vi "3DObjectBackground.vi"() -> ()   [LabVIEW 2011]
uses:
  <vilib>/picture/3D Picture Control/NI_3D Picture Control.lvlib
panel:
  out "3D Picture":refnum<vi>(3d-picture)
  in  "Angle":sgl
  in  "input cluster":T1
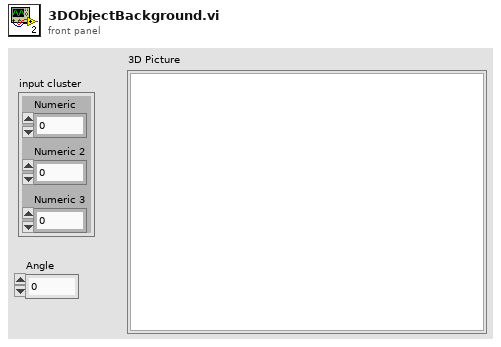
[diagram p1: front panel]
types:
  T1 = cluster{"Numeric":dbl, "Numeric 2":dbl, "Numeric 3":dbl}
  T2 = cluster{"number: 0 to 1":dbl, "number: 0 to 1":dbl, dbl, dbl}
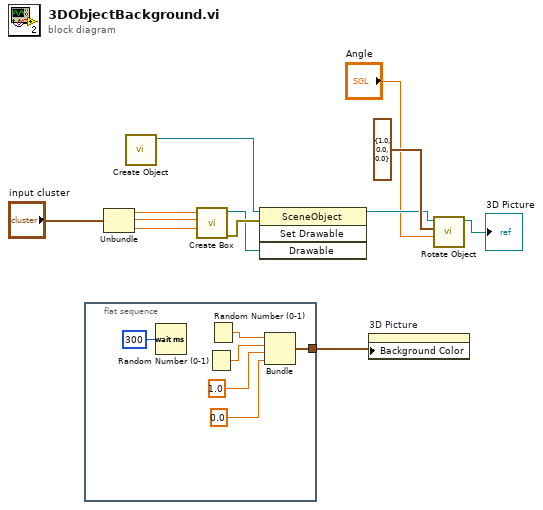
[diagram p0: block diagram]
diagram:
  n1 = flat-sequence {
    tunnel: [w13] -> w5
    frame #0 {
      n2 = Wait (ms)(milliseconds to wait=u32 300) -> ()  [unwired: 1 out]
      n3 = Random Number (0-1)() -> (number: 0 to 1=w16:dbl)
      n4 = Random Number (0-1)() -> (number: 0 to 1=w17:dbl)
      n5 = Bundle("number: 0 to 1"=w17, "number: 0 to 1"=w16, 1.0, 0.0) -> (w13:T2)  [unwired: 1 in]
    }
  }
  n6 = Unbundle("input cluster") -> ("Numeric"=w3:dbl, "Numeric 2"=w2:dbl, "Numeric 3"=w1:dbl)
  n7 = call <vilib>:"Create Object.vi"() -> ("Scene:New Object"=w11:refnum<vi>)  [unwired: 10 in, 1 out]
  n8 = call <vilib>:"Create Box.vi"("Length Z"=w1, "Length Y"=w2, "Length X"=w3) -> ("error out"=w12:errorcluster, "New Box Refnum"=w10:refnum<vi>)  [unwired: 7 in]
  n9 = invoke class="SceneObject" method="Set Drawable"(reference=w11, error in=w12, "Drawable"=w10) -> (reference out=w8:refnum<vi>)  [unwired: 1 in, 3 out]
  n10 = property on="3D Picture" class="SceneGraphDisp (strict)"("Background Color"=w5) -> ()  [unwired: 2 in, 2 out]
  n11 = call <vilib>:"Rotate Object.vi"("Angle"="Angle", "Axis"=cluster{"X":sgl, "Y":sgl, "Z":sgl} {"X"=1.0, "Y"=0.0, "Z"=0.0}, "Scene.Object In"=w8) -> ("Scene.Object Out"=→"3D Picture":refnum<vi>)  [unwired: 7 in, 1 out]
